vi "sub_SDR_rx_calcRxSamples.vi"(8 "Rx Parameters":T2={"IQ rate (Hz)"=4000000.0, "Carrier frequency [Hz]"=1187500000.0, "Gain [dB]"=10.0, "Antenna"="RX2", "Rx device name"="192.168.10.4; 192.168.10.5;"} {"Gain [dB]" format="%#_6f"; "Carrier frequency [Hz]" format="%#_6p"; "IQ rate (Hz)" format="%#_6p"}, 9 "decimating factor":i32, 10 "System options":T1={"Samples per symbol"=6, "Roll-Off"=0.75, "Filter length (symbols)"=7, "Modulation Type"=enum."64-QAM", "Payload Symbols"=1472, "Symbols per pilot"=6} {"Symbols per pilot" min=6 max=16 step=2; "Payload Symbols" min=16 max=8192 step=16; "Filter length (symbols)" min=1 max=9 step=2; "Roll-Off" min=0.0 max=1.0 step=0.01; "Samples per symbol" min=2 max=32 step=2}, 11 "Synch. Seq. Len":u16) -> (1 "Bit Rate [kbps]":dbl format="%#.1f", 2 "Performance":dbl, 3 "Numeric":i32)   [LabVIEW 2012]
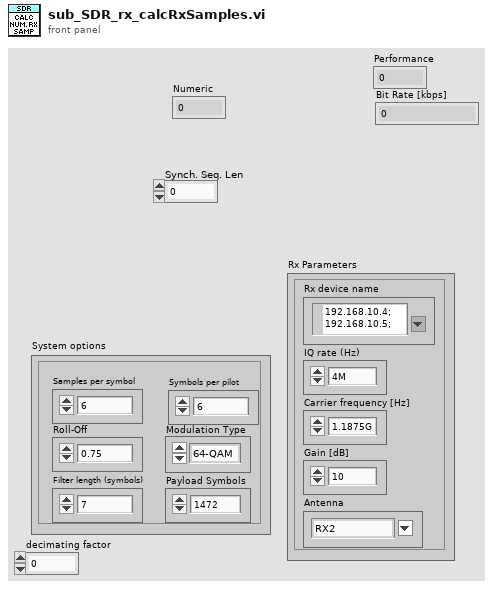
[diagram p1: front panel]
types:
  T1 = cluster{"Samples per symbol":i32, "Roll-Off":dbl, "Filter length (symbols)":i32, "Modulation Type":enum16{"BPSK", "4-QAM", "16-QAM", "64-QAM"}, "Payload Symbols":i32, "Symbols per pilot":i32}
  T2 = cluster{"IQ rate (Hz)":dbl, "Carrier frequency [Hz]":dbl, "Gain [dB]":dbl, "Antenna":string, "Rx device name":refnum<k15>}
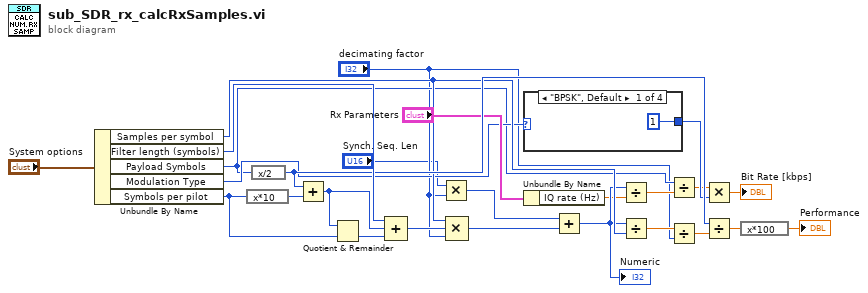
[diagram p0: block diagram]
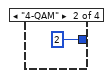
[diagram p2: hidden frame]
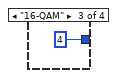
[diagram p3: hidden frame]
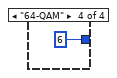
[diagram p4: hidden frame]
diagram:
  n1 = Unbundle By Name("System options") -> ("Samples per symbol"=w15:i32, "Filter length (symbols)"=w22:i32, "Payload Symbols"=w7:i32, "Modulation Type"=w8:enum16{"BPSK", "4-QAM", "16-QAM", "64-QAM"}, "Symbols per pilot"=w5:i32)
  n2 = expression code="x*10"(w5) -> (w25:i32)
  n3 = expression code="x/2"(w7) -> (w19:i32)
  n4 = Add(x=w19, y=w25) -> (x+y=w21:i32)
  n5 = Quotient & Remainder(x=w21, y=w5) -> (floor(x/y)=w26:i32)  [unwired: 1 out]
  n6 = Compound Arithmetic op=ADD(w22, w21, w26) -> (w24:i32)
  n7 = Multiply(x="Synch. Seq. Len", y="decimating factor") -> (x*y=w1:i32)
  n8 = Compound Arithmetic op=MULTIPLY(w15, w24, "decimating factor") -> (w23:i32)
  n9 = case shown="\"BPSK\", Default" w8 {
    tunnel: [1 2 4 6] -> w14
    frame "BPSK", Default {
    }
    frame "4-QAM" {
    }
    frame "16-QAM" {
    }
    frame "64-QAM" {
    }
  }
  n10 = Unbundle By Name("Rx Parameters") -> ("IQ rate (Hz)"=w11:dbl)
  n11 = Add(x=w1, y=w23) -> (x+y=w12:i32)
  "Numeric" <- w12
  n12 = Divide(x=w12, y=w11) -> (x/y=w10:dbl)
  n13 = Divide(x=w12, y=w15) -> (x/y=w20:dbl)
  n14 = Divide(x=w7, y=w10) -> (x/y=w9:dbl)
  n15 = Divide(x=w20, y="decimating factor") -> (x/y=w18:dbl)
  n16 = Multiply(x=w9, y=w14) -> (x*y=→"Bit Rate [kbps]":dbl)
  n17 = Divide(x=w19, y=w18) -> (x/y=w13:dbl)
  n18 = expression code="x*100"(w13) -> (→"Performance":dbl)
